vi "BRig_RT_comm_tcp_connect_HOSTwrite.vi"(8 "input_error":errorcluster) -> (0 "output_error":errorcluster, 2 "output_connected":bool, 3 "output_hTCP":refnum<k5>)   [LabVIEW 2014]
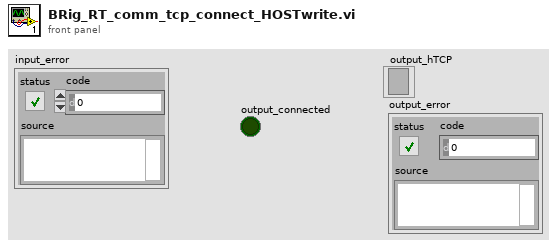
[diagram p1: front panel]
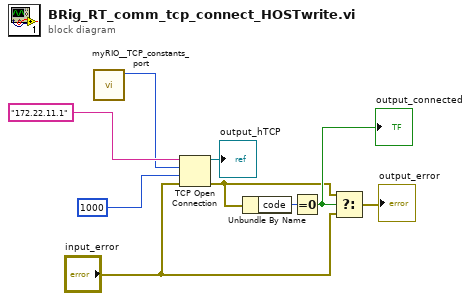
[diagram p0: block diagram]
diagram:
  n1 = call "myRIO__TCP_constants_port.vi"() -> ("output_TCP_port"=w1:u16)  [unwired: 11 in]
  n2 = TCP Open Connection(address="172.22.11.1" ("input_IP"), remote port or service name=w1, timeout ms (60000)=1000, error in (no error)="input_error") -> (connection ID=→"output_hTCP":refnum<k5>, error out=w5:errorcluster)  [unwired: 1 in]
  n3 = Unbundle By Name(w5) -> ("code"=w7:i32)
  n4 = Equal To 0?(x=w7) -> (x = 0?=w6:bool)
  "output_connected" <- w6
  n5 = Select(t=w5, s=w6, f="input_error") -> (s? t:f=→"output_error":errorcluster)
